vi "RT Driver VI.vi"(7 "Operation":T1, 11 "Device Reference in":T2 format="%.0x") -> (0 "Error Code":i32)   [LabVIEW 2021, in "DAQ Analog InOut Engine.lvlib"]
uses:
  DAQ Analog InOut Engine.lvlib
  <vilib>/NI VeriStand/Custom Device API/Custom Device Item Ref.ctl
  <vilib>/NI VeriStand/Custom Device API/Hardware Interface Driver VI Operation.ctl
  Shared/Compiled.Settings.ctl
  System Explorer/Types/Output Channel Parameters.ctl
  System Explorer/Types/Input Channel Parameters.ctl
  <vilib>/NI/NIVS Inline Async API/_VS Inline Async API/VS Inline Async API/VS Inline Async API.lvclass
  <vilib>/NI/NIVS Inline Async API/_VS Inline Async API/VS Inline Async API/VS Inline Async API.lvclass/VS Inline Async API.ctl
  <vilib>/NI/NIVS Inline Async API/_Data Access Engine/Data Access Engine/Data Access Engine.lvclass/Data Access Engine.ctl
  <vilib>/NI/NIVS Inline Async API/_Data Access Engine/Access Type Classes/Write/Write.lvclass/Write.ctl
  <vilib>/NI/NIVS Inline Async API/_Data Access Engine/Access Type Classes/ReadWrite/ReadWrite.lvclass/ReadWrite.ctl
  <vilib>/NI/NIVS Inline Async API/_Data Access Engine/Access Type Classes/Read/Read.lvclass/Read.ctl
  <vilib>/NI/NIVS Inline Async API/_Data Access Engine/Data Access Engine/Methods/Data.Engine.Read Data from HW.vi
  <vilib>/NI/NIVS Inline Async API/_VS Inline Async API/Error Handling Process/SubVIs/Error.GetError.vi
  <vilib>/NI/NIVS Inline Async API/_Data Access Engine/Data Access Engine/Methods/Data.Engine.Write Data to HW.vi
  <vilib>/NI/NIVS Inline Async API/_Data Access Engine/Access Type Classes/ReadWrite/ReadWrite.EngineData.vi
  <vilib>/NI/NIVS Inline Async API/_Data Access Engine/Access Type Classes/Write/Write.EngineData.vi
  <vilib>/NI/NIVS Inline Async API/_Data Access Engine/Access Type Classes/Read/Read.EngineData.vi
  <vilib>/NI VeriStand/Custom Device API/NI VeriStand - Get Channel Value by Data Reference.vi
  <vilib>/NI VeriStand/Custom Device API/NI VeriStand - Set Channel Value by Data Reference.vi
  <vilib>/NI VeriStand/Custom Device API/NI VeriStand - Get Channel Values by Block Data Reference.vi
  Shared/Constants.vi
  <vilib>/NI VeriStand/Custom Device API/Get Item Property (Variant).vi
  DAQ Analog Out.Async.vi
  DAQ Analog In.Async.vi
  <vilib>/NI VeriStand/Custom Device API/Global Data Refs.vi
  <vilib>/NI VeriStand/Custom Device API/Custom Device API.lvlib
  <vilib>/NI VeriStand/Custom Device Tools/Custom Device Utility Library/Custom Device Utility Library.lvlib
  Shared/DAQ Analog InOut Shared.lvlib
  System Explorer/DAQ Analog InOut System Explorer.lvlib
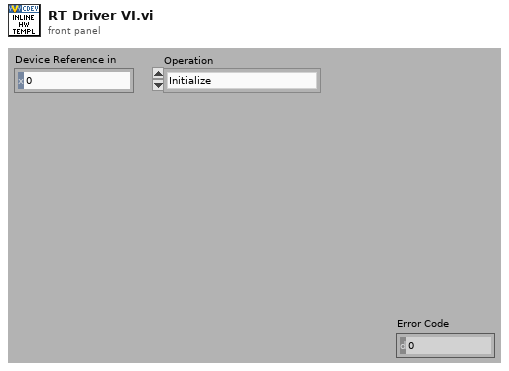
[diagram p1: front panel]
types:
  T1 = typedef "Custom Device API.lvlib/Hardware Interface Driver VI Operation.ctl" = enum16{"Initialize", "Start", "Read Data from HW", "Write Data to HW", "Close"}
  T2 = typedef "Custom Device API.lvlib/Custom Device Item Ref.ctl" = u64
  T3 = typedef "DAQ Analog InOut Shared.lvlib/Compiled.Settings.ctl" = cluster{"Name":string, "AO Enable":bool, "AI Enable":bool, "Main Page Parameters":cluster{"AI Channels Used":u8, "AO Channels Used":u8, "Select channel type to add":string, "Device Name in Max":string, "PCL Decimation":u16, "Async Timeout (ms)":u16}, "Output Channel Parameters":T4, "Input Channel Parameters":T5}
  T4 = typedef "DAQ Analog InOut System Explorer.lvlib/Output Channel Parameters.ctl" = cluster{"AO MaxV":dbl, "AO MinV":dbl}
  T5 = typedef "DAQ Analog InOut System Explorer.lvlib/Input Channel Parameters.ctl" = cluster{"AI MaxV":dbl, "AI MinV":dbl, "AI Sample Rate":dbl, "Input Configuration":u16}
  T6 = cluster{"Async":refnum<class "VS Inline Async API.lvclass">, "Compiled.Settings":T3}
  T7 = typedef "DAQ Analog InOut Engine.lvlib/AO Properties.ctl" = cluster{"AO Channels List":string, "Output Channel Parameters":T4}
  T8 = typedef "DAQ Analog InOut Engine.lvlib/AI Properties.ctl" = cluster{"AI Channels List":string, "Input Channel Parameters":T5}
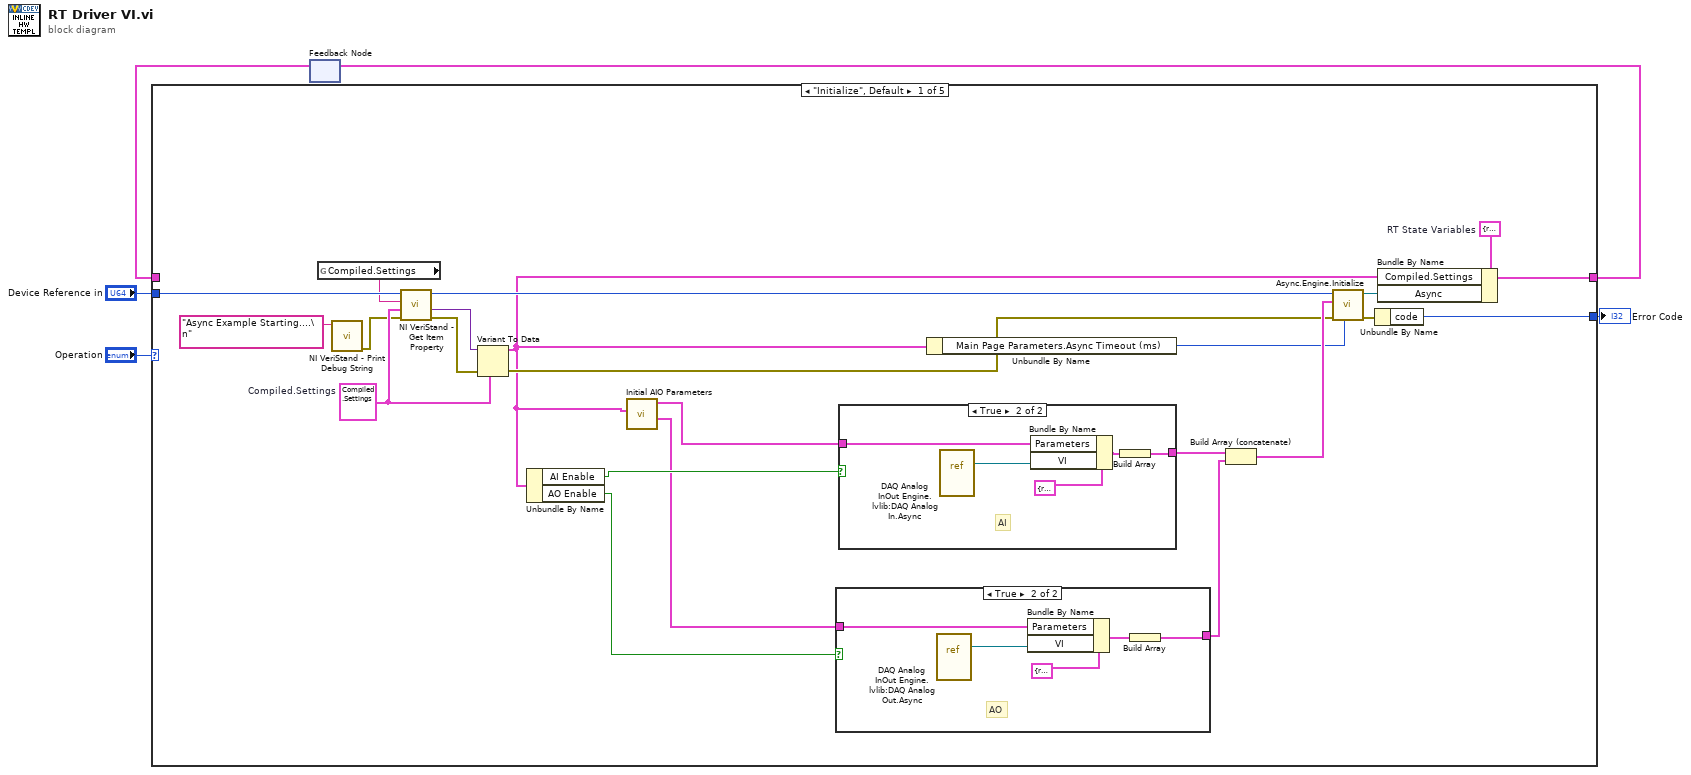
[diagram p0: block diagram]
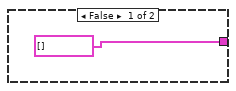
[diagram p2: hidden frame]
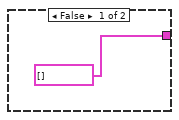
[diagram p3: hidden frame]
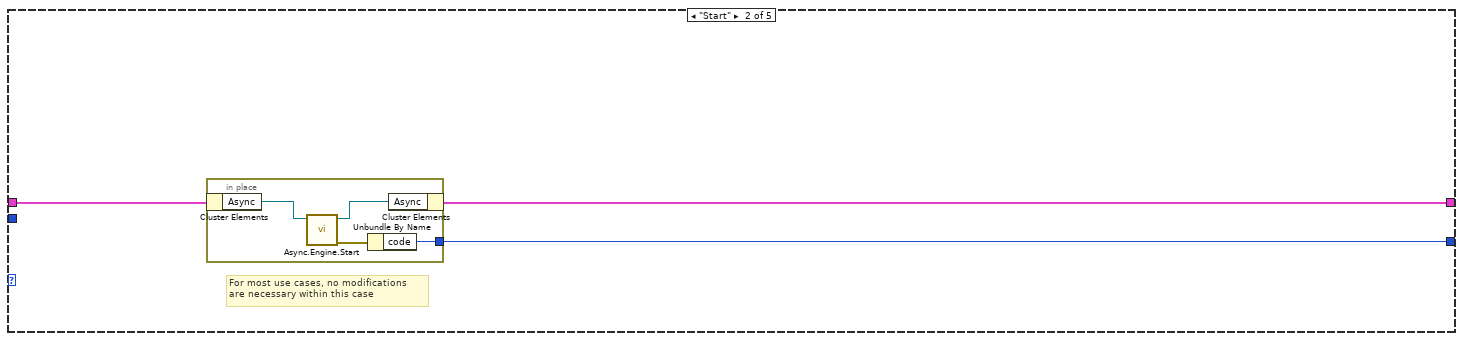
[diagram p4: hidden frame]
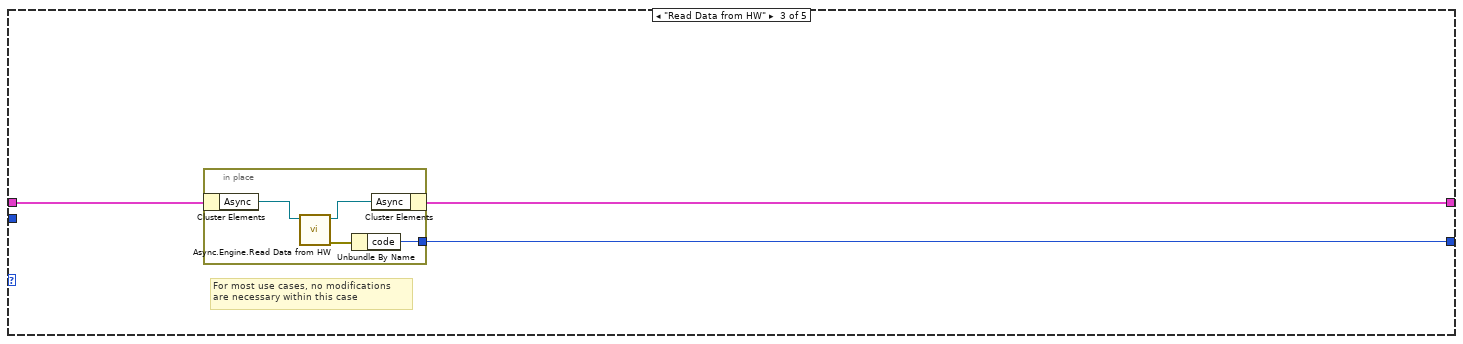
[diagram p5: hidden frame]
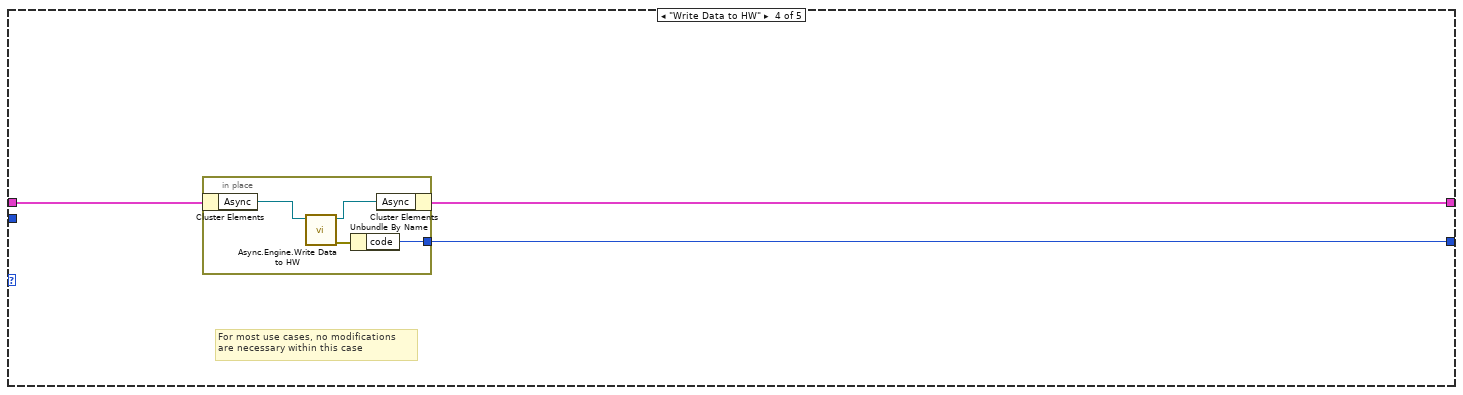
[diagram p6: hidden frame]
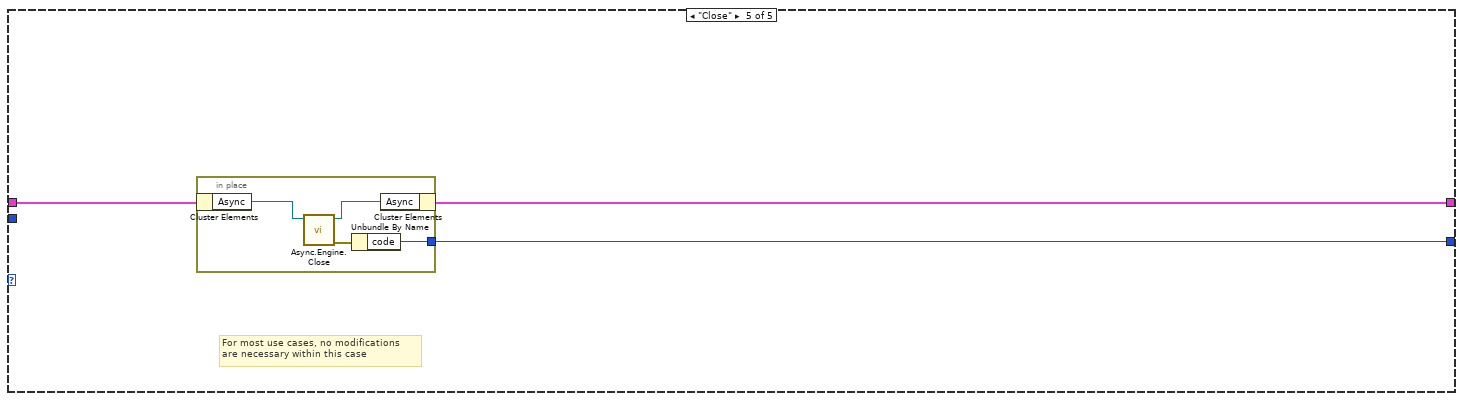
[diagram p7: hidden frame]
diagram:
  n1 = feedback #1() -> (w3:T6)  [unwired: 1 out]
  n2 = case shown="\"Initialize\", Default" "Operation" {
    tunnel: [w26 w42 w48 w55 w63] -> w4
    tunnel: w3 -> [_ w43 w50 w56 w64]
    tunnel: "Device Reference in" -> [w24 _ _ _ _]
    tunnel: [w28 w41 w49 w57 w62] -> w1
    frame "Initialize", Default {
      w18 = T6 {"Async"=refnum, "Compiled.Settings"={"Name"="", "AO Enable"=FALSE, "AI Enable"=FALSE, "Main Page Parameters"={"AI Channels Used"=0, "AO Channels Used"=0, "Select channel type to add"="", "Device Name in Max"="PXI1Slot2", "PCL Decimation"=0, "Async Timeout (ms)"=0}, "Output Channel Parameters"={"AO MaxV"=0.0, "AO MinV"=0.0}, "Input Channel Parameters"={"AI MaxV"=0.0, "AI MinV"=0.0, "AI Sample Rate"=0.0, "Input Configuration"=10083}}}  # RT State Variables
      w19 = T3 {"Name"="", "AO Enable"=FALSE, "AI Enable"=FALSE, "Main Page Parameters"={"AI Channels Used"=0, "AO Channels Used"=0, "Select channel type to add"="", "Device Name in Max"="PXI1Slot2", "PCL Decimation"=0, "Async Timeout (ms)"=0}, "Output Channel Parameters"={"AO MaxV"=0.0, "AO MinV"=0.0}, "Input Channel Parameters"={"AI MaxV"=0.0, "AI MinV"=0.0, "AI Sample Rate"=0.0, "Input Configuration"=10083}}  # Compiled.Settings
      n3 = global read "Constants.vi" "Compiled.Settings"() -> (w21:string)
      n4 = call <vilib>:"NI VeriStand - Print Debug String.vi"("Message"="Async Example Starting....\n") -> ("error out"=w14:errorcluster)  [unwired: 10 in]
      n5 = call-poly <vilib>:"NI VeriStand - Get Item Property.vi"("error in (no error)"=w14, "Default Value"=w19, "Property Name"=w21, "Item Ref in"=w24) -> ("error out"=w23:errorcluster, "Value"=w22:variant, "Item Ref out"=w15:T2)  [unwired: 4 in, 1 out]
      n6 = Variant To Data(error in=w23, type=w19, Variant=w22) -> (data=w8:T3, error out=w16:errorcluster)
      n7 = Unbundle By Name(w8) -> ("AI Enable"=w11:bool, "AO Enable"=w9:bool)
      n8 = call "Initial AIO Parameters.vi"("Compiled.Settings"=w8) -> ("AO Properties"=w6:T7, "AI Properties"=w7:T8)  [unwired: 9 in]
      n9 = case shown="True" w9 {
        tunnel: [cluster{"VI":refnum<vi>, "Parameters":variant}[] [] w30] -> w10
        tunnel: w6 -> [_ w32]
        frame False {
        }
        frame True {
          # "AO"
          n10 = vi-ref "DAQ Analog InOut Engine.lvlib:DAQ Analog Out.Async.vi"() -> (w33:refnum<vi>)
          n11 = Bundle By Name(cluster=cluster{"VI":refnum<vi>, "Parameters":variant} {"VI"=refnum, "Parameters"=variant} ("Process"), "Parameters"=w32, "VI"=w33) -> (w31:cluster{"VI":refnum<vi>, "Parameters":variant})
          n12 = Build Array(w31) -> (w30:cluster{"VI":refnum<vi>, "Parameters":variant}[])
        }
      }
      n13 = case shown="True" w11 {
        tunnel: [cluster{"VI":refnum<vi>, "Parameters":variant}[] [] w36] -> w25
        tunnel: w7 -> [_ w38]
        frame False {
        }
        frame True {
          # "AI"
          n14 = vi-ref "DAQ Analog InOut Engine.lvlib:DAQ Analog In.Async.vi"() -> (w39:refnum<vi>)
          n15 = Bundle By Name(cluster=cluster{"VI":refnum<vi>, "Parameters":variant} {"VI"=refnum, "Parameters"=variant} ("Process"), "Parameters"=w38, "VI"=w39) -> (w37:cluster{"VI":refnum<vi>, "Parameters":variant})
          n16 = Build Array(w37) -> (w36:cluster{"VI":refnum<vi>, "Parameters":variant}[])
        }
      }
      n17 = Unbundle By Name(w8) -> ("Main Page Parameters.Async Timeout (ms)"=w12:u16)
      n18 = Build Array (concatenate)(w25, w10) -> (w17:cluster{"VI":refnum<vi>, "Parameters":variant}[])
      n19 = call <vilib>:"Async.Engine.Initialize.vi"("Timeout (ms) (5000)"=w12, "error in (no error)"=w16, "Processes"=w17, "Custom Device Ref"=w15) -> ("error out"=w20:errorcluster, "Async"=w27:refnum<class "VS Inline Async API.lvclass">)  [unwired: 6 in]
      n20 = Unbundle By Name(w20) -> ("code"=w28:i32)
      n21 = Bundle By Name(cluster=w18, "Compiled.Settings"=w8, "Async"=w27) -> (w26:T6)
    }
    frame "Start" {
      # "For most use cases, no modifications \nare necessary within this case"
      n22 = in-place {
        in-place-border: [w44] -> w41
        n23 = in-place-cluster #2(w43) -> ("Async"=w47:refnum<class "VS Inline Async API.lvclass">)
        n24 = call <vilib>:"Async.Engine.Start.vi"("VS Inline Async API in"=w47) -> ("error out"=w45:errorcluster, "VS Inline Async API out"=w46:refnum<class "VS Inline Async API.lvclass">)  [unwired: 9 in]
        n25 = Unbundle By Name(w45) -> ("code"=w44:i32)
        n26 = in-place-cluster #2("Async"=w46) -> (w42:T6)
      }
    }
    frame "Read Data from HW" {
      # "For most use cases, no modifications \nare necessary within this case"
      n27 = in-place {
        in-place-border: [w52] -> w49
        n28 = in-place-cluster #3(w50) -> ("Async"=w54:refnum<class "VS Inline Async API.lvclass">)
        n29 = call <vilib>:"Async.Engine.Read Data from HW.vi"("Async in"=w54) -> ("error out"=w51:errorcluster, "Async out"=w53:refnum<class "VS Inline Async API.lvclass">)  [unwired: 9 in]
        n30 = Unbundle By Name(w51) -> ("code"=w52:i32)
        n31 = in-place-cluster #3("Async"=w53) -> (w48:T6)
      }
    }
    frame "Write Data to HW" {
      # "For most use cases, no modifications \nare necessary within this case"
      n32 = in-place {
        in-place-border: [w61] -> w57
        n33 = in-place-cluster #4(w56) -> ("Async"=w59:refnum<class "VS Inline Async API.lvclass">)
        n34 = call <vilib>:"Async.Engine.Write Data to HW.vi"("VS Inline Async API in"=w59) -> ("error out"=w60:errorcluster, "VS Inline Async API out"=w58:refnum<class "VS Inline Async API.lvclass">)  [unwired: 9 in]
        n35 = Unbundle By Name(w60) -> ("code"=w61:i32)
        n36 = in-place-cluster #4("Async"=w58) -> (w55:T6)
      }
    }
    frame "Close" {
      # "For most use cases, no modifications \nare necessary within this case"
      n37 = in-place {
        in-place-border: [w66] -> w62
        n38 = in-place-cluster #5(w64) -> ("Async"=w68:refnum<class "VS Inline Async API.lvclass">)
        n39 = call <vilib>:"Async.Engine.Close.vi"("Async in"=w68) -> ("error out"=w65:errorcluster, "Async out"=w67:refnum<class "VS Inline Async API.lvclass">)  [unwired: 9 in]
        n40 = Unbundle By Name(w65) -> ("code"=w66:i32)
        n41 = in-place-cluster #5("Async"=w67) -> (w63:T6)
      }
    }
  }
  "Error Code" <- w1
  n42 = feedback-in #1(w4) -> ()
